vi "Handle Message.vi"(5 "Stack ID":u8, 7 "Function ID":u8, 8 "error in (no error)":errorcluster, 10 "Data":string, 11 "Barometer Bricklet in":refnum<class "Barometer Bricklet.lvclass">) -> (0 "error out":errorcluster, 1 "Send Answer":bool, 2 "Answer":variant, 3 "Barometer Bricklet out":refnum<class "Barometer Bricklet.lvclass">)   [LabVIEW 2011, in "Tinkerforge.lvlib" / "Barometer Bricklet.lvclass"]
doc: "This VI is the child implementation of \"Handle Message.vi\" and processes all responses for this device type."
uses:
  Barometer Bricklet.lvclass
  Barometer Bricklet.lvclass/Barometer Bricklet.ctl
  Device/Device.lvclass
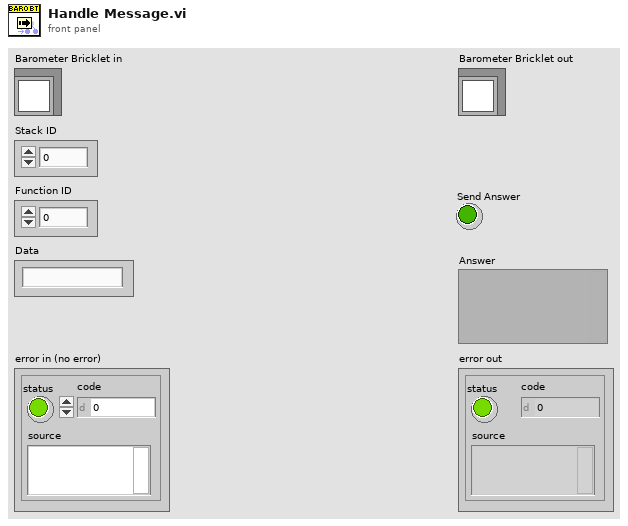
[diagram p1: front panel]
types:
  T1 = typedef "Tinkerforge.lvlib/Barometer Bricklet.lvclass/Callback Threshold.ctl" = cluster{"Callback Option":T2, "min":i32, "max":i32}
  T2 = typedef "Tinkerforge.lvlib/Device.lvclass/Callback Option.ctl" = enum8{"CB off", "outside range", "inside range", "smaller", "greater"}
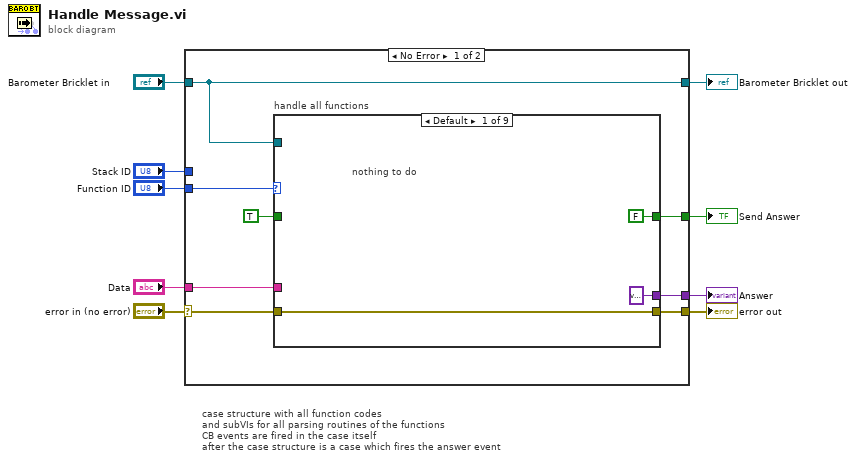
[diagram p0: block diagram]
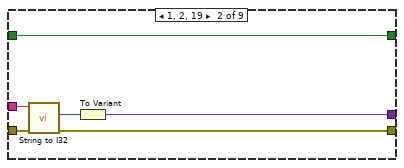
[diagram p2: hidden frame]
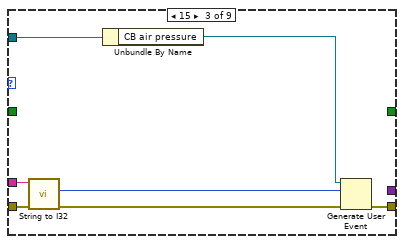
[diagram p3: hidden frame]
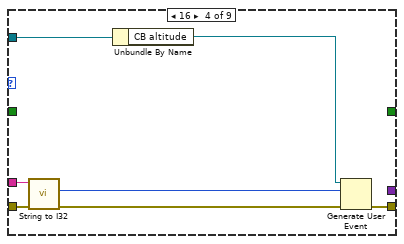
[diagram p4: hidden frame]
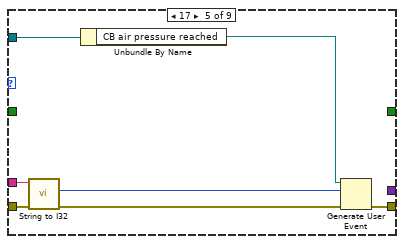
[diagram p5: hidden frame]
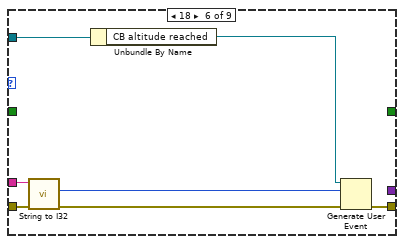
[diagram p6: hidden frame]
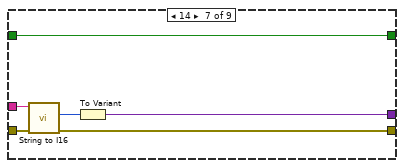
[diagram p7: hidden frame]
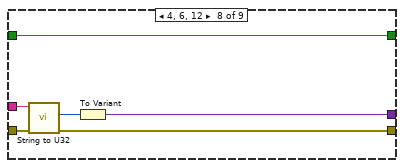
[diagram p8: hidden frame]
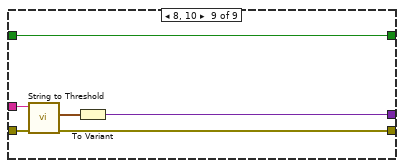
[diagram p9: hidden frame]
diagram:
  # "case structure with all function codes\nand subVIs for all parsing routines of the functions\nCB events are fired in the case itself\nafter the case structure is a case which fires the answer event"
  n1 = case shown="No Error" "error in (no error)" {
    selector: "error in (no error)" -> [w14 w73]
    tunnel: "Barometer Bricklet in" -> [w17 w74]
    tunnel: "Stack ID" -> [_ _]
    tunnel: "Function ID" -> [w16 _]
    tunnel: "Data" -> [w13 _]
    tunnel: [w17 w74] -> w4
    tunnel: [w12 w73] -> w3
    tunnel: [w11 _] -> w2
    tunnel: [w10 _] -> w1
    frame No Error {
      n2 = case "handle all functions" shown="Default" w16 {
        tunnel: w14 -> [w20 w26 w33 w40 w47 w54 w60 w66 w69]
        tunnel: TRUE -> [_ w23 _ _ _ _ w57 w63 w72]
        tunnel: [FALSE w23 _ _ _ _ w57 w63 w72] -> w10
        tunnel: [w20 w24 w30 w37 w44 w51 w58 w64 w68] -> w12
        tunnel: [variant ("Variant") w21 _ _ _ _ w55 w61 w71] -> w11
        tunnel: w17 -> [_ _ w29 w36 w43 w50 _ _ _]
        tunnel: w13 -> [_ w25 w32 w39 w46 w53 w59 w65 w70]
        frame Default {
          # "nothing to do"
        }
        frame 1, 2, 19 {
          n3 = call "String to I32.vi"("Error In"=w26, "String"=w25) -> ("Error Out"=w24:errorcluster, "I32"=w22:i32)  [unwired: 7 in, 1 out]
          n4 = To Variant(anything=w22) -> (Variant=w21:variant)
        }
        frame 15 {
          n5 = call "String to I32.vi"("Error In"=w33, "String"=w32) -> ("Error Out"=w31:errorcluster, "I32"=w27:i32)  [unwired: 7 in, 1 out]
          n6 = Unbundle By Name(w29) -> ("CB air pressure"=w28:refnum<user-event>)
          n7 = Generate User Event(user event=w28, event data cluster=w27, error in=w31) -> (error out=w30:errorcluster)  [unwired: 1 out]
        }
        frame 16 {
          n8 = call "String to I32.vi"("Error In"=w40, "String"=w39) -> ("Error Out"=w38:errorcluster, "I32"=w34:i32)  [unwired: 7 in, 1 out]
          n9 = Unbundle By Name(w36) -> ("CB altitude"=w35:refnum<user-event>)
          n10 = Generate User Event(user event=w35, event data cluster=w34, error in=w38) -> (error out=w37:errorcluster)  [unwired: 1 out]
        }
        frame 17 {
          n11 = call "String to I32.vi"("Error In"=w47, "String"=w46) -> ("Error Out"=w45:errorcluster, "I32"=w41:i32)  [unwired: 7 in, 1 out]
          n12 = Unbundle By Name(w43) -> ("CB air pressure reached"=w42:refnum<user-event>)
          n13 = Generate User Event(user event=w42, event data cluster=w41, error in=w45) -> (error out=w44:errorcluster)  [unwired: 1 out]
        }
        frame 18 {
          n14 = call "String to I32.vi"("Error In"=w54, "String"=w53) -> ("Error Out"=w52:errorcluster, "I32"=w48:i32)  [unwired: 7 in, 1 out]
          n15 = Unbundle By Name(w50) -> ("CB altitude reached"=w49:refnum<user-event>)
          n16 = Generate User Event(user event=w49, event data cluster=w48, error in=w52) -> (error out=w51:errorcluster)  [unwired: 1 out]
        }
        frame 14 {
          n17 = call "String to I16.vi"("Error In"=w60, "String"=w59) -> ("Error Out"=w58:errorcluster, "I16"=w56:i16)  [unwired: 7 in, 1 out]
          n18 = To Variant(anything=w56) -> (Variant=w55:variant)
        }
        frame 4, 6, 12 {
          n19 = call "String to U32.vi"("Error In"=w66, "String"=w65) -> ("Error Out"=w64:errorcluster, "U32"=w62:u32)  [unwired: 7 in, 1 out]
          n20 = To Variant(anything=w62) -> (Variant=w61:variant)
        }
        frame 8, 10 {
          n21 = call "String to Threshold.vi"("Error In"=w69, "String"=w70) -> ("Error Out"=w68:errorcluster, "Callback Threshold"=w67:T1)  [unwired: 7 in, 1 out]
          n22 = To Variant(anything=w67) -> (Variant=w71:variant)
        }
      }
    }
    frame Error {
    }
  }
  "error out" <- w3
  "Barometer Bricklet out" <- w4
  "Answer" <- w2
  "Send Answer" <- w1
